vi "GetBoolFromBoolCtrl.vi"(11 "bool ref":refnum<vi>) -> (3 "result":bool)   [LabVIEW 2018, in "Library-Ctrl.lvlib"]
uses:
  Library-Ctrl.lvlib
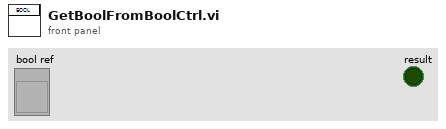
[diagram p1: front panel]
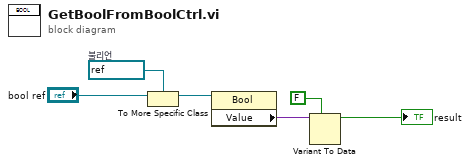
[diagram p0: block diagram]
diagram:
  w5 = refnum<vi> refnum  # 불리언
  n1 = To More Specific Class(target class=w5, reference="bool ref") -> (specific class reference=w4:refnum<vi>)  [unwired: 1 in, 1 out]
  n2 = property class="Bool"(reference=w4) -> ("Value"=w3:variant)  [unwired: 1 in, 2 out]
  n3 = Variant To Data(type=FALSE, Variant=w3) -> (data=→"result":bool)  [unwired: 1 in, 1 out]
